vi "Data Store.vi"(8 "error in (no error)":errorcluster, 9 "Data File":path, 10 "Contact in":T1[](array[typedef]), 11 "Command":T8=enum."Load") -> (0 "error out":errorcluster, 2 "Data Modified?":bool, 3 "Contacts out":T1[](array[typedef]))   [LabVIEW 2014, in "Contact Data.lvlib"]
doc: "The main action engine VI that stores the address book data using functional global variables."
uses:
  Contact Data.lvlib
  Contact.ctl
  Position.ctl
  Controls.ctl
  DestinationCluster.ctl
  DesinationControls.ctl
  PathData.ctl
  Components/PathFinder/Controls/PathControl.ctl
  Command.ctl
  File Data.ctl
  <vilib>/Utility/xml.llb/Read From XML File(string).vi
  <vilib>/Utility/xml.llb/Write to XML File(string).vi
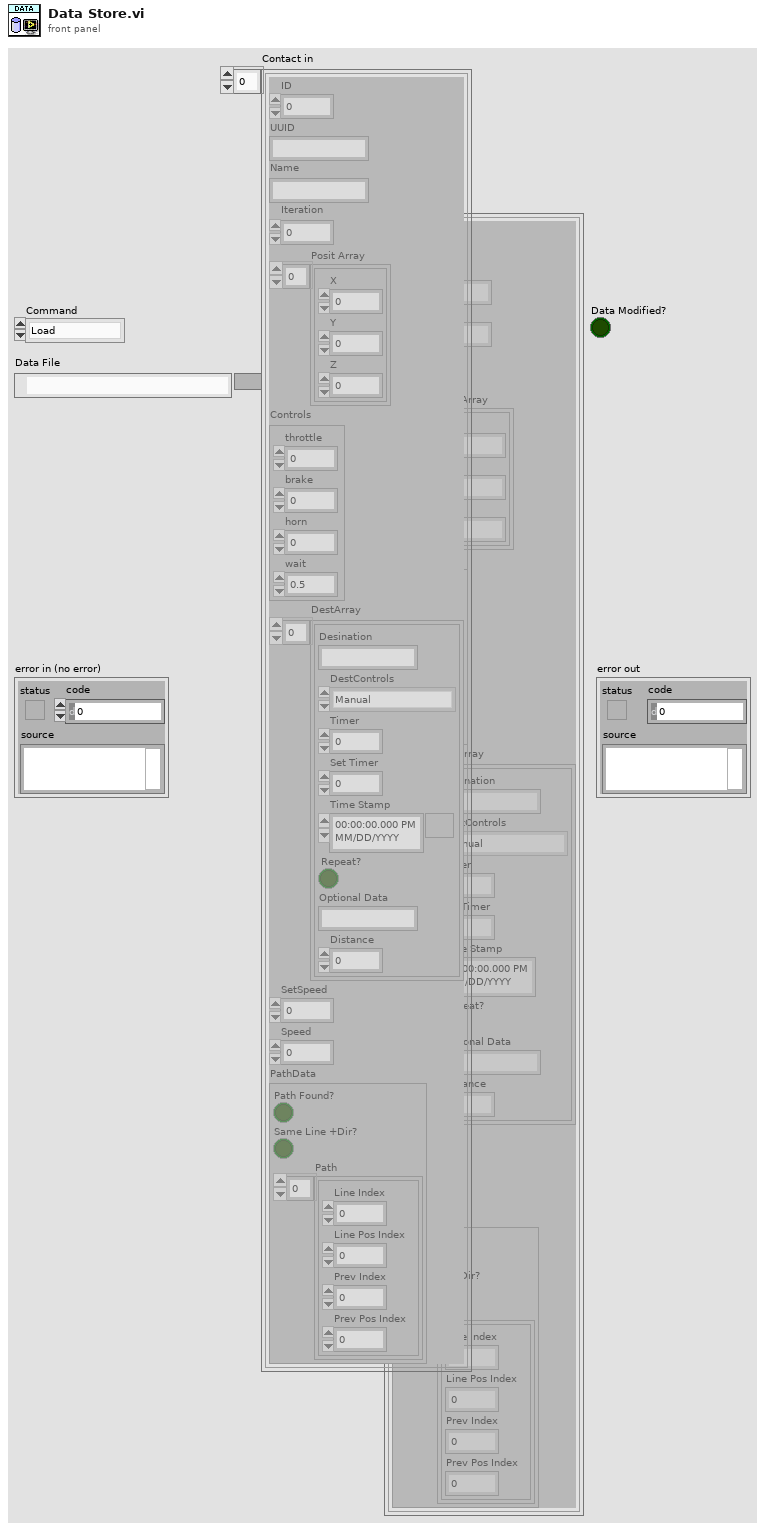
[diagram p1: front panel]
types:
  T1 = typedef "Contact Data.lvlib/Contact.ctl" = cluster{"ID":u32, "UUID":string, "Name":string, "Iteration":i32, "Posit Array":T2[], "Controls":T3, "DestArray":T4[], "SetSpeed":dbl, "Speed":dbl, "PathData":T6}
  T2 = typedef "Contact Data.lvlib/Position.ctl" = cluster{"X":dbl, "Y":dbl, "Z":dbl}
  T3 = typedef "Contact Data.lvlib/Controls.ctl" = cluster{"throttle":dbl, "brake":dbl, "horn":dbl, "wait":dbl}
  T4 = typedef "Contact Data.lvlib/DestinationCluster.ctl" = cluster{"Desination":string, "DestControls":T5, "Timer":u32, "Set Timer":u32, "Time Stamp":timestamp, "Repeat?":bool, "Optional Data":string, "Distance":dbl}
  T5 = typedef "Contact Data.lvlib/DesinationControls.ctl" = enum16{"Tracker", "Manual", "Stop", "Station DateTime", "Station Timer", "Maintain"}
  T6 = typedef "Contact Data.lvlib/PathData.ctl" = cluster{"Path Found?":bool, "Same Line +Dir?":bool, "Path":T7[]}
  T7 = typedef "PathControl.ctl" = cluster{"Line Index":i32, "Line Pos Index ":i32, "Prev Index ":i32, "Prev Pos Index":i32}
  T8 = typedef "Contact Data.lvlib/Command.ctl" = enum16{"Set All Contacts", "Load", "Save", "Get All Data", "Get Single Data (ID)", "Get Single Data", "Set Position", "Set Single Path", "Set Destinations", "Set Controls", "Remove Single Data", "Remove UUID Contact", "Set Single ALL", "Is Data Modified", "Import Data"}
  T9 = typedef "Contact Data.lvlib/File Data.ctl" = cluster{"Last ID":u32, "Contacts":T1[]}
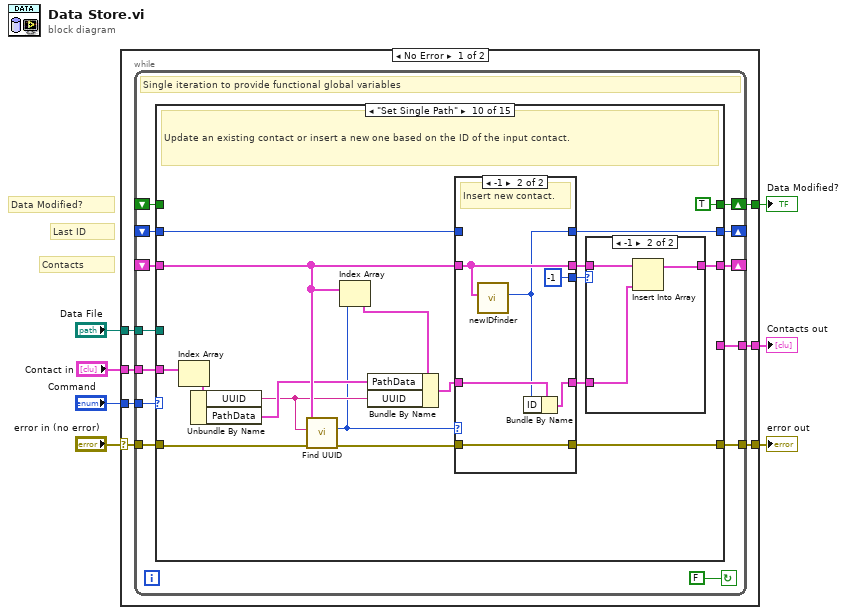
[diagram p0: block diagram]
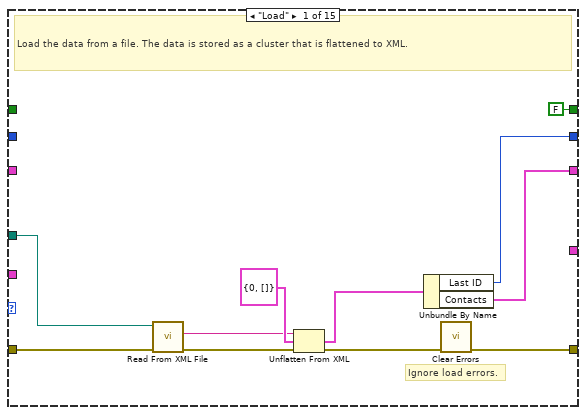
[diagram p2: hidden frame]
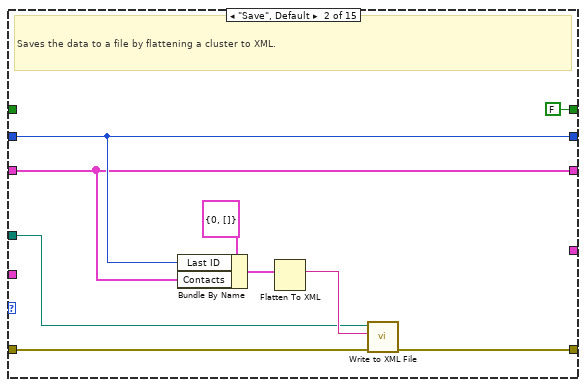
[diagram p3: hidden frame]
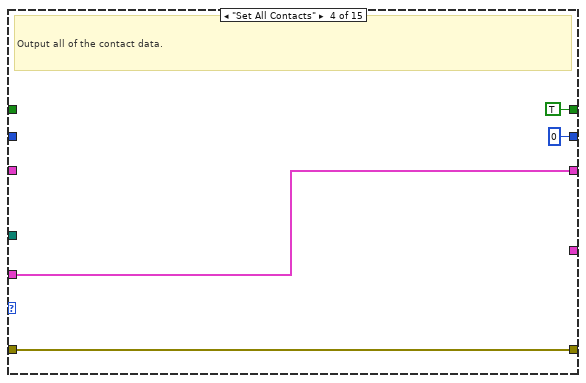
[diagram p5: hidden frame]
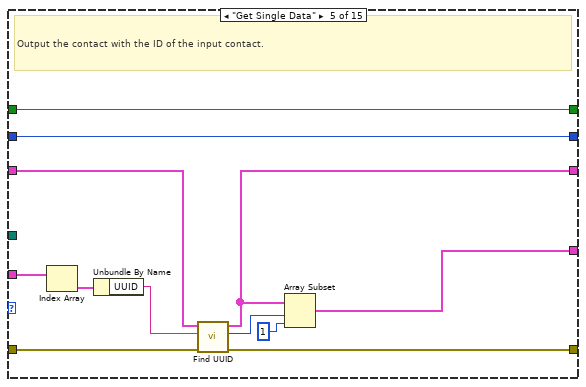
[diagram p6: hidden frame]
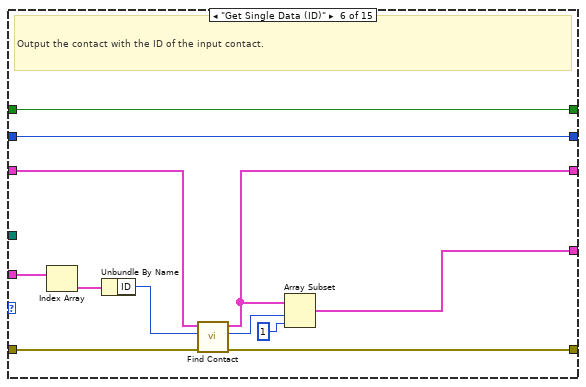
[diagram p7: hidden frame]
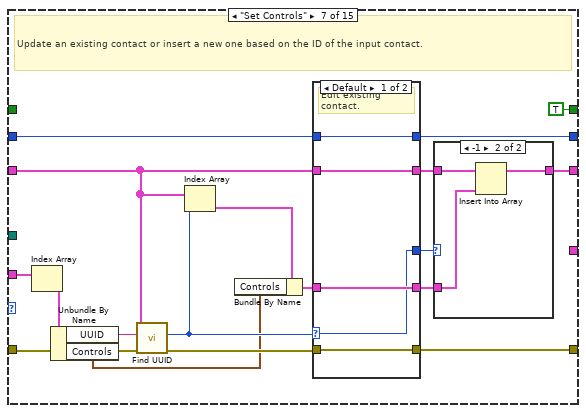
[diagram p8: hidden frame]
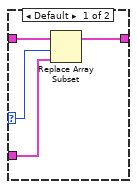
[diagram p9: hidden frame]
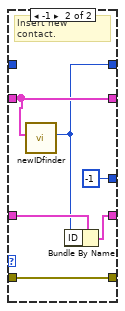
[diagram p10: hidden frame]
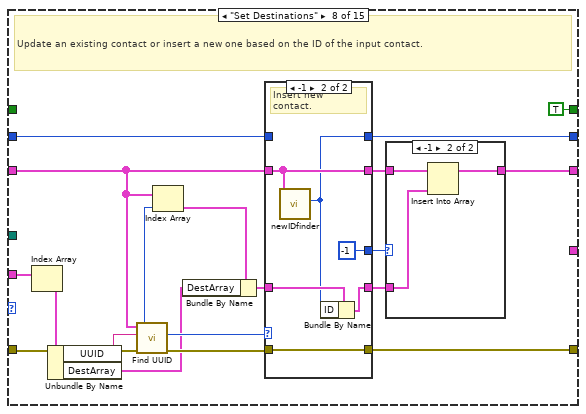
[diagram p11: hidden frame]
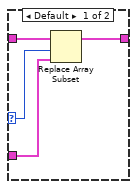
[diagram p12: hidden frame]
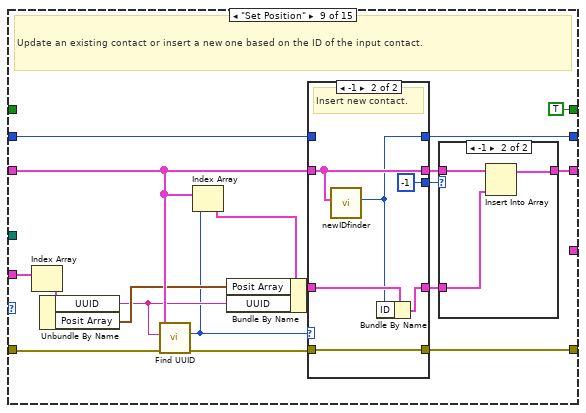
[diagram p14: hidden frame]
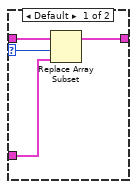
[diagram p15: hidden frame]
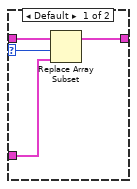
[diagram p17: hidden frame]
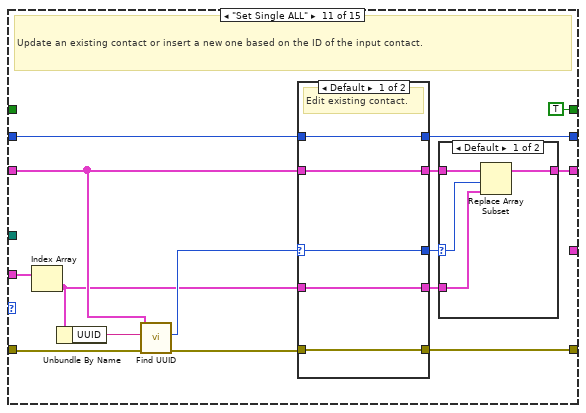
[diagram p19: hidden frame]
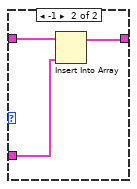
[diagram p20: hidden frame]
diagram:
  # "Contacts"
  # "Last ID"
  # "Data Modified?"
  n1 = case shown="No Error" "error in (no error)" {
    selector: "error in (no error)" -> [w13 w297]
    tunnel: [w14 w297] -> w7
    tunnel: "Command" -> [w12 _]
    tunnel: "Contact in" -> [w11 _]
    tunnel: [w10 _] -> w4
    tunnel: "Data File" -> [w9 _]
    tunnel: [w8 _] -> w2
    frame No Error {
      n2 = while {
        tunnel: [w26] -> w14
        tunnel: w13 -> [w25]
        tunnel: w12 -> [w22]
        tunnel: w11 -> [w15]
        shift-right: [w27] -> _
        shift-left: _ -> [w20]
        shift-right: [w23] -> _
        shift-left: _ -> [w24]
        tunnel: [w19] -> w10
        shift-right: [w18] -> w8
        shift-left: _ -> [w17]
        tunnel: w9 -> [w16]
        stop <- FALSE continue-if-true
        # "Single iteration to provide functional global variables"
        n3 = case shown="\"Set Single Path\"" w22 {
          tunnel: w25 -> [w35 w44 w50 w55 w67 w79 w87 w123 w160 w196 w230 w261 w276 w287 w296]
          tunnel: [w28 w43 w50 w55 w62 w74 w91 w127 w163 w199 w232 w260 w275 w287 w296] -> w26
          tunnel: w20 -> [_ w40 w49 _ w66 w78 w82 w118 w156 w192 w227 w267 w282 w290 w293]
          tunnel: [w32 w40 w49 w54 w65 w77 w95 w131 w167 w203 w236 w264 w279 w290 w294] -> w27
          tunnel: w15 -> [_ _ _ w54 w57 w69 w90 w126 w162 w198 w231 w259 w274 _ w292]
          tunnel: w24 -> [_ w41 w51 _ w63 w75 w86 w122 w159 w195 w229 w263 w278 w289 w291]
          tunnel: [w33 w41 w51 u32 0 ("Last ID") w63 w75 w93 w129 w165 w201 w234 w263 w278 w289 w291] -> w23
          tunnel: [FALSE FALSE w48 TRUE w61 w73 TRUE TRUE TRUE TRUE TRUE TRUE TRUE w288 w295] -> w18
          tunnel: [_ _ w49 _ w60 w72 _ _ _ _ _ _ _ _ w292] -> w19
          tunnel: w17 -> [_ _ w48 _ w61 w73 _ _ _ _ _ _ _ w288 w295]
          tunnel: w16 -> [w31 w42 _ _ _ _ _ _ _ _ _ _ _ _ _]
          frame "Load" {
            # "Ignore load errors."
            # "Load the data from a file. The data is stored as a cluster that is flattened to XML."
            n4 = call-poly <vilib>:"Read From XML File.vi"("error in (no error)"=w35, "XML File Path"=w31) -> ("error out"=w29:errorcluster, "XML Elements"=w30:string)  [unwired: 7 in, 1 out]
            n5 = Unflatten From XML(xml string=w30, type=T9 {"Last ID"=0, "Contacts"=[]} ("Data"), error in (no error)=w29) -> (value=w36:T9, error out=w34:errorcluster)
            n6 = Unbundle By Name(w36) -> ("Last ID"=w33:u32, "Contacts"=w32:T1[])
            n7 = call <vilib>:"Clear Errors.vi"("error in (no error)"=w34) -> ("error out"=w28:errorcluster)  [unwired: 5 in, 1 out]
          }
          frame "Save", Default {
            # "Saves the data to a file by flattening a cluster to XML."
            n8 = Bundle By Name(cluster=T9 {"Last ID"=0, "Contacts"=[]} ("File Data"), "Last ID"=w41, "Contacts"=w40) -> (w45:T9)
            n9 = Flatten To XML(anything=w45) -> (xml string=w47:string)
            n10 = call-poly <vilib>:"Write to XML File.vi"("error in (no error)"=w44, "XML Input"=w47, "XML File Path"=w42) -> ("error out"=w43:errorcluster)  [unwired: 6 in, 2 out]
          }
          frame "Get All Data" {
            # "Output all of the contact data."
          }
          frame "Set All Contacts" {
            # "Output all of the contact data."
          }
          frame "Get Single Data" {
            # "Output the contact with the ID of the input contact."
            n11 = Index Array(array=w57) -> (element=w58:T1)  [unwired: 1 in]
            n12 = Unbundle By Name(w58) -> ("UUID"=w56:string)
            n13 = call "Find UUID.vi"("error in (no error)"=w67, "ID"=w56, "Data"=w66) -> ("error out"=w62:errorcluster, "Index"=w64:i32, "dup Data"=w65:T1[])  [unwired: 6 in]
            n14 = Array Subset(array=w65, index=w64, length=1) -> (w60:T1[])
          }
          frame "Get Single Data (ID)" {
            # "Output the contact with the ID of the input contact."
            n15 = Index Array(array=w69) -> (element=w70:T1)  [unwired: 1 in]
            n16 = Unbundle By Name(w70) -> ("ID"=w68:u32)
            n17 = call "Find Contact.vi"("error in (no error)"=w79, "ID"=w68, "Data"=w78) -> ("error out"=w74:errorcluster, "Index"=w76:i32, "dup Data"=w77:T1[])  [unwired: 6 in]
            n18 = Array Subset(array=w77, index=w76, length=1) -> (w72:T1[])
          }
          frame "Set Controls" {
            # "Update an existing contact or insert a new one based on the ID of the input contact."
            n19 = Index Array(array=w90) -> (element=w85:T1)  [unwired: 1 in]
            n20 = Unbundle By Name(w85) -> ("UUID"=w89:string, "Controls"=w80:T3)
            n21 = call "Find UUID.vi"("error in (no error)"=w87, "ID"=w89, "Data"=w82) -> ("error out"=w88:errorcluster, "Index"=w83:i32)  [unwired: 6 in, 1 out]
            n22 = Index Array(array=w82, index=w83) -> (element=w81:T1)
            n23 = Bundle By Name(cluster=w81, "Controls"=w80) -> (w84:T1)
            n24 = case shown="Default" w83 {
              selector: w83 -> [w105 _]
              tunnel: w82 -> [w107 w111]
              tunnel: w88 -> [w106 w115]
              tunnel: [w107 w111] -> w96
              tunnel: [w105 -1 ("Index")] -> w97
              tunnel: [w106 w115] -> w91
              tunnel: w86 -> [w108 _]
              tunnel: w84 -> [w109 w113]
              tunnel: [w109 w112] -> w94
              tunnel: [w108 w110] -> w93
              frame Default {
                # "Edit existing contact."
              }
              frame -1 {
                # "Insert new contact."
                n25 = call "newIDfinder.vi"("dup Data"=w111) -> ("ID"=w110:u32)  [unwired: 10 in]
                n26 = Bundle By Name(cluster=w113, "ID"=w110) -> (w112:T1)
              }
            }
            n27 = case shown="-1" w97 {
              selector: w97 -> [w99 _]
              tunnel: w96 -> [w101 w104]
              tunnel: w94 -> [w100 w103]
              tunnel: [w98 w102] -> w95
              frame Default {
                n28 = Replace Array Subset "Replace Array Subset"(array=w101, new element=w100, index=w99) -> (w98:T1[])
              }
              frame -1 {
                n29 = Insert Into Array "Insert Into Array"(array=w104, new element=w103) -> (w102:T1[])  [unwired: 1 in]
              }
            }
          }
          frame "Set Destinations" {
            # "Update an existing contact or insert a new one based on the ID of the input contact."
            n30 = Index Array(array=w126) -> (element=w121:T1)  [unwired: 1 in]
            n31 = Unbundle By Name(w121) -> ("UUID"=w125:string, "DestArray"=w116:T4[])
            n32 = call "Find UUID.vi"("error in (no error)"=w123, "ID"=w125, "Data"=w118) -> ("error out"=w124:errorcluster, "Index"=w119:i32)  [unwired: 6 in, 1 out]
            n33 = Index Array(array=w118, index=w119) -> (element=w117:T1)
            n34 = Bundle By Name(cluster=w117, "DestArray"=w116) -> (w120:T1)
            n35 = case shown="-1" w119 {
              selector: w119 -> [w143 _]
              tunnel: w118 -> [w141 w147]
              tunnel: w124 -> [w142 w151]
              tunnel: [w141 w147] -> w132
              tunnel: [w143 -1 ("Index")] -> w133
              tunnel: [w142 w151] -> w127
              tunnel: w122 -> [w144 _]
              tunnel: w120 -> [w145 w149]
              tunnel: [w145 w148] -> w130
              tunnel: [w144 w146] -> w129
              frame Default {
                # "Edit existing contact."
              }
              frame -1 {
                # "Insert new contact."
                n36 = call "newIDfinder.vi"("dup Data"=w147) -> ("ID"=w146:u32)  [unwired: 10 in]
                n37 = Bundle By Name(cluster=w149, "ID"=w146) -> (w148:T1)
              }
            }
            n38 = case shown="-1" w133 {
              selector: w133 -> [w135 _]
              tunnel: w132 -> [w137 w140]
              tunnel: w130 -> [w136 w139]
              tunnel: [w134 w138] -> w131
              frame Default {
                n39 = Replace Array Subset "Replace Array Subset"(array=w137, new element=w136, index=w135) -> (w134:T1[])
              }
              frame -1 {
                n40 = Insert Into Array "Insert Into Array"(array=w140, new element=w139) -> (w138:T1[])  [unwired: 1 in]
              }
            }
          }
          frame "Set Position" {
            # "Update an existing contact or insert a new one based on the ID of the input contact."
            n41 = Index Array(array=w162) -> (element=w158:T1)  [unwired: 1 in]
            n42 = Unbundle By Name(w158) -> ("UUID"=w153:string, "Posit Array"=w154:T2[])
            n43 = call "Find UUID.vi"("error in (no error)"=w160, "ID"=w153, "Data"=w156) -> ("error out"=w161:errorcluster, "Index"=w152:i32)  [unwired: 6 in, 1 out]
            n44 = Index Array(array=w156, index=w152) -> (element=w155:T1)
            n45 = Bundle By Name(cluster=w155, "Posit Array"=w154, "UUID"=w153) -> (w157:T1)
            n46 = case shown="-1" w152 {
              selector: w152 -> [w179 _]
              tunnel: w156 -> [w177 w183]
              tunnel: w161 -> [w178 w187]
              tunnel: [w177 w183] -> w168
              tunnel: [w179 -1 ("Index")] -> w169
              tunnel: [w178 w187] -> w163
              tunnel: w159 -> [w180 _]
              tunnel: w157 -> [w181 w185]
              tunnel: [w181 w184] -> w166
              tunnel: [w180 w182] -> w165
              frame Default {
                # "Edit existing contact."
              }
              frame -1 {
                # "Insert new contact."
                n47 = call "newIDfinder.vi"("dup Data"=w183) -> ("ID"=w182:u32)  [unwired: 10 in]
                n48 = Bundle By Name(cluster=w185, "ID"=w182) -> (w184:T1)
              }
            }
            n49 = case shown="-1" w169 {
              selector: w169 -> [w171 _]
              tunnel: w168 -> [w173 w176]
              tunnel: w166 -> [w172 w174]
              tunnel: [w170 w175] -> w167
              frame Default {
                n50 = Replace Array Subset "Replace Array Subset"(array=w173, new element=w172, index=w171) -> (w170:T1[])
              }
              frame -1 {
                n51 = Insert Into Array "Insert Into Array"(array=w176, new element=w174) -> (w175:T1[])  [unwired: 1 in]
              }
            }
          }
          frame "Set Single Path" {
            # "Update an existing contact or insert a new one based on the ID of the input contact."
            n52 = Index Array(array=w198) -> (element=w194:T1)  [unwired: 1 in]
            n53 = Unbundle By Name(w194) -> ("UUID"=w189:string, "PathData"=w190:T6)
            n54 = call "Find UUID.vi"("error in (no error)"=w196, "ID"=w189, "Data"=w192) -> ("error out"=w197:errorcluster, "Index"=w188:i32)  [unwired: 6 in, 1 out]
            n55 = Index Array(array=w192, index=w188) -> (element=w191:T1)
            n56 = Bundle By Name(cluster=w191, "PathData"=w190, "UUID"=w189) -> (w193:T1)
            n57 = case shown="-1" w188 {
              selector: w188 -> [w215 _]
              tunnel: w192 -> [w213 w219]
              tunnel: w197 -> [w214 w223]
              tunnel: [w213 w219] -> w204
              tunnel: [w215 -1 ("Index")] -> w205
              tunnel: [w214 w223] -> w199
              tunnel: w195 -> [w216 _]
              tunnel: w193 -> [w217 w221]
              tunnel: [w217 w220] -> w202
              tunnel: [w216 w218] -> w201
              frame Default {
                # "Edit existing contact."
              }
              frame -1 {
                # "Insert new contact."
                n58 = call "newIDfinder.vi"("dup Data"=w219) -> ("ID"=w218:u32)  [unwired: 10 in]
                n59 = Bundle By Name(cluster=w221, "ID"=w218) -> (w220:T1)
              }
            }
            n60 = case shown="-1" w205 {
              selector: w205 -> [w207 _]
              tunnel: w204 -> [w209 w212]
              tunnel: w202 -> [w208 w210]
              tunnel: [w206 w211] -> w203
              frame Default {
                n61 = Replace Array Subset "Replace Array Subset"(array=w209, new element=w208, index=w207) -> (w206:T1[])
              }
              frame -1 {
                n62 = Insert Into Array "Insert Into Array"(array=w212, new element=w210) -> (w211:T1[])  [unwired: 1 in]
              }
            }
          }
          frame "Set Single ALL" {
            # "Update an existing contact or insert a new one based on the ID of the input contact."
            n63 = Index Array(array=w231) -> (element=w224:T1)  [unwired: 1 in]
            n64 = Unbundle By Name(w224) -> ("UUID"=w225:string)
            n65 = call "Find UUID.vi"("error in (no error)"=w230, "ID"=w225, "Data"=w227) -> ("error out"=w226:errorcluster, "Index"=w228:i32)  [unwired: 6 in, 1 out]
            n66 = case shown="Default" w228 {
              selector: w228 -> [w248 _]
              tunnel: w227 -> [w246 w252]
              tunnel: w226 -> [w247 w256]
              tunnel: [w246 w252] -> w237
              tunnel: [w248 -1 ("Index")] -> w238
              tunnel: [w247 w256] -> w232
              tunnel: w229 -> [w249 _]
              tunnel: w224 -> [w250 w254]
              tunnel: [w250 w253] -> w235
              tunnel: [w249 w251] -> w234
              frame Default {
                # "Edit existing contact."
              }
              frame -1 {
                # "Insert new contact."
                n67 = call "newIDfinder.vi"("dup Data"=w252) -> ("ID"=w251:u32)  [unwired: 10 in]
                n68 = Bundle By Name(cluster=w254, "ID"=w251) -> (w253:T1)
              }
            }
            n69 = case shown="Default" w238 {
              selector: w238 -> [w240 _]
              tunnel: w237 -> [w242 w245]
              tunnel: w235 -> [w241 w243]
              tunnel: [w239 w244] -> w236
              frame Default {
                n70 = Replace Array Subset "Replace Array Subset"(array=w242, new element=w241, index=w240) -> (w239:T1[])
              }
              frame -1 {
                n71 = Insert Into Array "Insert Into Array"(array=w245, new element=w243) -> (w244:T1[])  [unwired: 1 in]
              }
            }
          }
          frame "Remove Single Data" {
            # "Remove a contact from the data using the ID of the input contact."
            n72 = Index Array(array=w259) -> (element=w257:T1)  [unwired: 1 in]
            n73 = Unbundle By Name(w257) -> ("ID"=w258:u32)
            n74 = call "Find Contact.vi"("error in (no error)"=w261, "ID"=w258, "Data"=w267) -> ("error out"=w260:errorcluster, "Index"=w265:i32, "dup Data"=w266:T1[])  [unwired: 6 in]
            n75 = case shown="Default" w265 {
              selector: w265 -> [_ w270]
              tunnel: w266 -> [w268 w271]
              tunnel: [w268 w269] -> w264
              frame -1 {
              }
              frame Default {
                n76 = Delete From Array(array=w271, index=w270) -> (array with subset deleted=w269:T1[])  [unwired: 1 in, 1 out]
              }
            }
          }
          frame "Remove UUID Contact" {
            # "Remove a contact from the data using the ID of the input contact."
            n77 = Index Array(array=w274) -> (element=w272:T1)  [unwired: 1 in]
            n78 = Unbundle By Name(w272) -> ("UUID"=w273:string)
            n79 = call "Find UUID.vi"("error in (no error)"=w276, "ID"=w273, "Data"=w282) -> ("error out"=w275:errorcluster, "Index"=w280:i32, "dup Data"=w281:T1[])  [unwired: 6 in]
            n80 = case shown="Default" w280 {
              selector: w280 -> [_ w285]
              tunnel: w281 -> [w283 w286]
              tunnel: [w283 w284] -> w279
              frame -1 {
              }
              frame Default {
                n81 = Delete From Array(array=w286, index=w285) -> (array with subset deleted=w284:T1[])  [unwired: 1 in, 1 out]
              }
            }
          }
          frame "Is Data Modified" {
            # "Output if the data has been modified or not since the last save command."
          }
          frame "Import Data" {
            # "Insert all of the input contacts, replacing the IDs of each one."
            n82 = Insert Into Array(array=w293, new element=w292) -> (w294:T1[])  [unwired: 1 in]
          }
        }
      }
    }
    frame Error {
    }
  }
  "Contacts out" <- w4
  "error out" <- w7
  "Data Modified?" <- w2
